vi "Top level UI-Shortcut menus handler.vi"(11 "ItemTag":string) -> ()   [LabVIEW 2013]
uses:
  Windows/System config window/Typedefs/HW Setup tab control.ctl
  Global Variables/gl_UI Ctrl Refs.vi
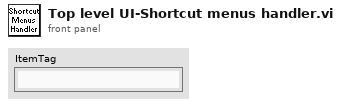
[diagram p1: front panel]
types:
  T1 = typedef "HW Setup tab control.ctl" = enum32{"Control system ", "Triggers", "DAQ FPGA", "HW Channels Setup", "XY stage", "Encoder", "System Setup", "Cameras", "AOL Properties", "Calibration Settings", "Reserved 1", "Reserved 2"}
  T2 = typedef "UI ctrl refs cluster.ctl" = cluster{"Top level VI path":path, "Top level VI ref":refnum<vi>, "User menu ref":refnum<k9>, "Sub Panel control":refnum<vi>, "Imaging Param Tab":refnum<vi>, "Occurrence-Start drivers":refnum<k4>, "Occurrence-Speed logging initialised":refnum<k4>, "Occurrence-XYZ stage initialised":refnum<k4>, "Exit button":refnum<vi>, "Status ind":refnum<vi>, "Return to Origin":refnum<vi>, "Speed Logging":refnum<vi>, "Time Lapse":refnum<vi>, "Live Imaging":refnum<vi>, "AOL Z Stack":refnum<vi>, "Motor Z Stack":refnum<vi>, "Funct Acq button":refnum<vi>, "Hard Shutter":refnum<vi>, "Virtual Shutter":refnum<vi>, "Laser Power":refnum<vi>, "AOL Mode":refnum<vi>, "Frame Size":refnum<vi>, "Field of View":refnum<vi>, "Dwell Time":refnum<vi>, "Zoom":refnum<vi>, "AOL Z":refnum<vi>, "Objective":refnum<vi>, "Axis":refnum<vi>, "Paths & Names":refnum<vi>, "Experiment folder path (ind.)":refnum<vi>, "Last State (Ind.)":refnum<vi>, "Laser wavelength ind (nm)":refnum<vi>, "Averages":refnum<vi>, "Angle (degrees)":refnum<vi>, "X centre":refnum<vi>, "Y centre":refnum<vi>, "Plane Mode":refnum<vi>, "# Planes":refnum<vi>, "Z Start":refnum<vi>, "Z Stop":refnum<vi>, "Z Step":refnum<vi>, "PMT 1":refnum<vi>, "PMT 2":refnum<vi>, "Stage XYZ Position":refnum<vi>, "Pockels@Z Start":refnum<vi>, "Pockels@Z Stop":refnum<vi>, "Obtain Z Start":refnum<vi>, "Obtain Z Stop":refnum<vi>, "Live stim.trig.period":refnum<vi>, "Live stim.trig.enable":refnum<vi>, "Funct. Acq. Pockels Modulation":refnum<vi>, "Enable Video Recording":refnum<vi>, "Video Record-Live Imaging":refnum<vi>, "Video Record-Funct acq":refnum<vi>, "AOL Z-stack Chirps Ready (ind)":refnum<vi>, "Center freq ind (nm)":refnum<vi>, "Logging queue (ind)":refnum<vi>, "Back aperture power (ind.)":refnum<vi>, "Power after objective (ind.)":refnum<vi>, "Switch user":refnum<vi>}
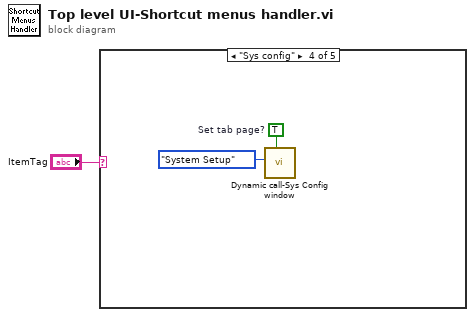
[diagram p0: block diagram]
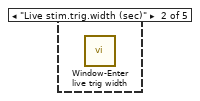
[diagram p3: hidden frame]
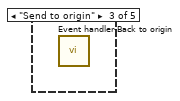
[diagram p4: hidden frame]
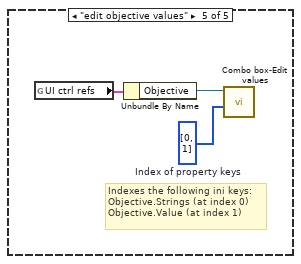
[diagram p5: hidden frame]
diagram:
  n1 = case shown="\"Sys config\"" "ItemTag" {
    frame Default {
    }
    frame "Live stim.trig.width (sec)" {
      n2 = call "Window-Enter live trig width.vi"() -> ()  [unwired: 11 in, 1 out]
    }
    frame "Send to origin" {
      n3 = call "Event handler-Back to origin.vi"() -> ()  [unwired: 12 in]
    }
    frame "Sys config" {
      w2 = TRUE  # Set tab page?
      n4 = call "Dynamic call-Sys Config window.vi"("Set tab page? (F)"=w2, "System Config Tab Control"=HW_Setup_tab_control."System Setup") -> ()  [unwired: 9 in, 1 out]
    }
    frame "edit objective values" {
      w4 = i32[] [0, 1]  # Index of property keys
      # "Indexes the following ini keys:\nObjective.Strings (at index 0)\nObjective.Value (at index 1)"
      n5 = global read "gl_UI Ctrl Refs.vi" "UI ctrl refs"() -> (w6:T2)
      n6 = Unbundle By Name(w6) -> ("Objective"=w5:refnum<vi>)
      n7 = call "Combo box-Edit values.vi"("Index of property key"=w4, "Combo box ref"=w5) -> ()  [unwired: 10 in]
    }
  }
